vi "Format Table.vi"(8 "button":bool, 9 "clear":bool, 10 "BotPose":cluster{"X":dbl, "Y":dbl}, 11 "Insta360 Pose":cluster{"X":dbl, "Y":dbl}) -> (0 "Points Info for Plot":cluster{dbl[], dbl[], dbl[], dbl[]}, 1 "BoolText.Text":string, 2 "Numeric out":sgl, 3 "Array":string[][](array[string]))   [LabVIEW 2025]
uses:
  d5bf1515-77e7-4290-83ff-5f447d93a6cc.vi
  <vilib>/vision/NI_Vision_Development_Module.lvlib
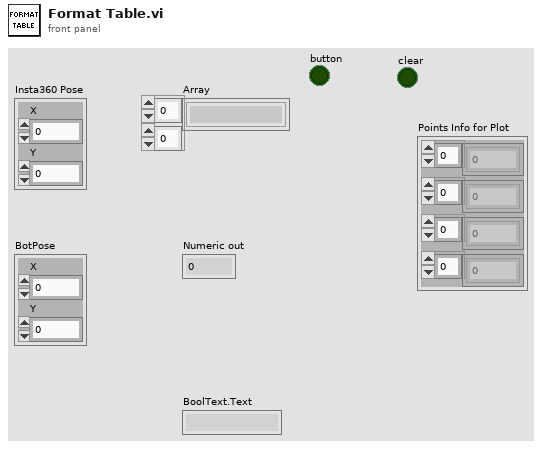
[diagram p1: front panel]
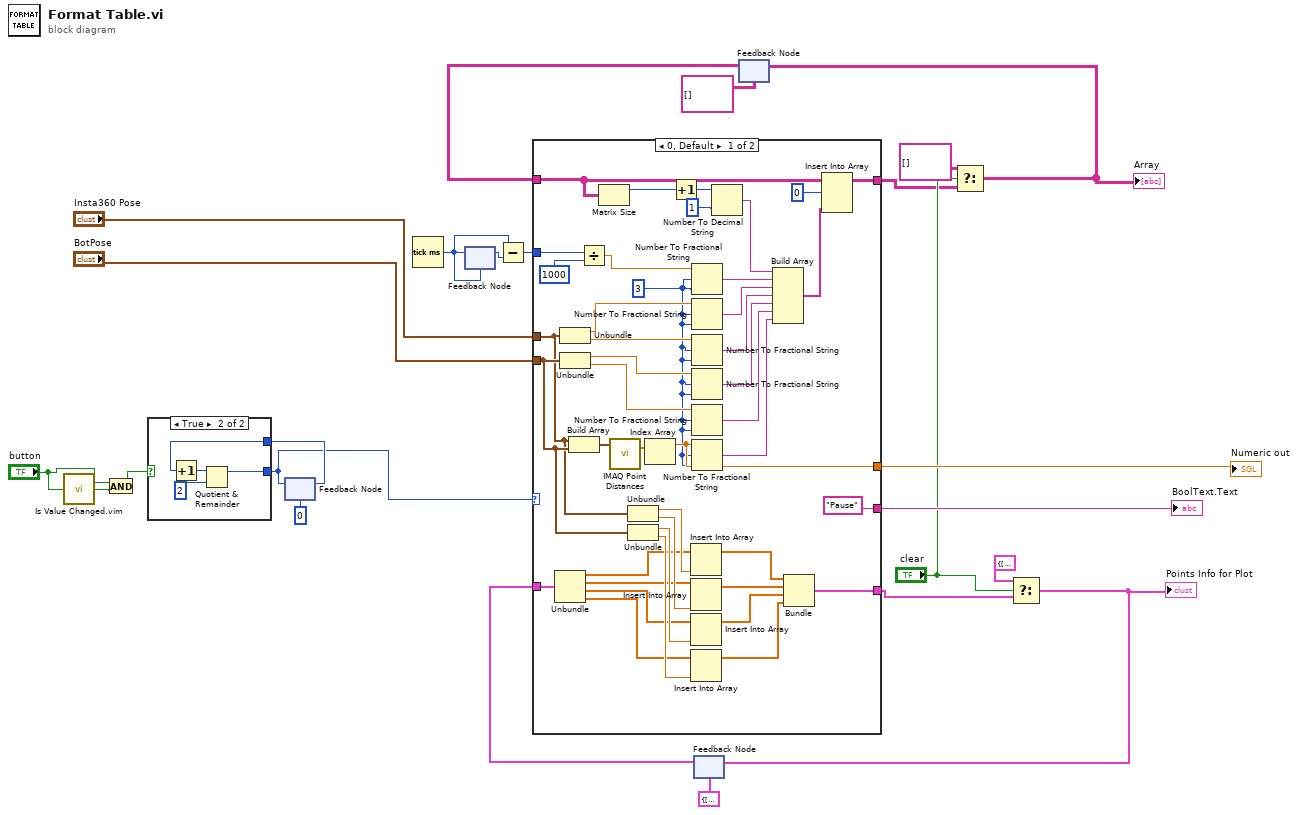
[diagram p0: block diagram]
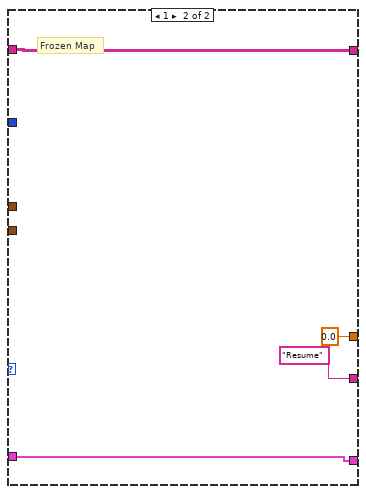
[diagram p3: hidden frame]
diagram:
  n1 = call "Is Value Changed.vim"("value"="button") -> ("changed or first call?"=w15:bool)
  n2 = And(x="button", y=w15) -> (x .and. y?=w16:bool)
  n3 = feedback #1(u16 0) -> (w17:u16)
  n4 = case shown="True" w16 {
    tunnel: w17 -> [w25 w29]
    tunnel: [w25 w26] -> w14
    frame False {
    }
    frame True {
      n5 = Increment(x=w29) -> (x+1=w28:u16)
      n6 = Quotient & Remainder(x=w28, y=u16 2) -> (x-y*floor(x/y)=w26:u16)  [unwired: 1 out]
    }
  }
  n7 = feedback-in #1(w14) -> ()
  n8 = Tick Count (ms)() -> (millisecond timer value=w2:u32)
  n9 = feedback-in #2(w2) -> ()
  n10 = feedback #2(w2) -> (w1:u32)
  n11 = Subtract(x=w2, y=w1) -> (x-y=w3:u32)
  n12 = feedback #3(cluster{dbl[], dbl[], dbl[], dbl[]} {[], [], [], []}) -> (w12:cluster{dbl[], dbl[], dbl[], dbl[]})
  n13 = feedback #4(string[][] []) -> (w21:string[][])
  n14 = case shown="0, Default" w14 {
    tunnel: ["Pause" ("BoolText.Text") "Resume" ("BoolText.Text")] -> w19
    tunnel: w3 -> [w32 _]
    tunnel: w21 -> [w70 w74]
    tunnel: [w64 w74] -> w6
    tunnel: "Insta360 Pose" -> [w47 _]
    tunnel: "BotPose" -> [w48 _]
    tunnel: [w52 sgl 0.0] -> w22
    tunnel: [w38 w72] -> w10
    tunnel: w12 -> [w37 w72]
    frame 0, Default {
      w51 = i16 3 ("width (-)")
      n15 = Unbundle(w37) -> (w36:dbl[], w35:dbl[], w34:dbl[], w33:dbl[])
      n16 = Unbundle(w47) -> ("X"=w63:dbl, "Y"=w62:dbl)
      n17 = Unbundle(w48) -> ("X"=w61:dbl, "Y"=w60:dbl)
      n18 = Build Array(w47, w48) -> (w59:cluster{"X":dbl, "Y":dbl}[])
      n19 = Divide(x=w32, y=u32 1000) -> (x/y=w30:dbl)
      n20 = Matrix Size(0:w70) -> (1:w69:i32)  [unwired: 1 out]
      n21 = call "IMAQ Point Distances"("Points"=w59) -> ("Distances"=w53:sgl[])  [unwired: 4 in, 1 out]
      n22 = Unbundle(w47) -> ("X"=w43:dbl, "Y"=w44:dbl)
      n23 = Unbundle(w48) -> ("X"=w45:dbl, "Y"=w46:dbl)
      n24 = Index Array(array=w53) -> (element=w52:sgl)  [unwired: 1 in]
      n25 = Increment(x=w69) -> (x+1=w50:i32)
      n26 = Insert Into Array(array=w36, new element=w43) -> (w42:dbl[])  [unwired: 1 in]
      n27 = Insert Into Array(array=w35, new element=w44) -> (w41:dbl[])  [unwired: 1 in]
      n28 = Insert Into Array(array=w34, new element=w45) -> (w40:dbl[])  [unwired: 1 in]
      n29 = Insert Into Array(array=w33, new element=w46) -> (w39:dbl[])  [unwired: 1 in]
      n30 = Number To Fractional String(number=w30, width (-)=w51, precision (6)=w51) -> (F-format string=w68:string)  [unwired: 1 in]
      n31 = Number To Fractional String(number=w63, width (-)=w51, precision (6)=w51) -> (F-format string=w58:string)  [unwired: 1 in]
      n32 = Number To Fractional String(number=w62, width (-)=w51, precision (6)=w51) -> (F-format string=w57:string)  [unwired: 1 in]
      n33 = Number To Fractional String(number=w61, width (-)=w51, precision (6)=w51) -> (F-format string=w56:string)  [unwired: 1 in]
      n34 = Number To Fractional String(number=w60, width (-)=w51, precision (6)=w51) -> (F-format string=w55:string)  [unwired: 1 in]
      n35 = Number To Fractional String(number=w52, width (-)=w51, precision (6)=w51) -> (F-format string=w54:string)  [unwired: 1 in]
      n36 = Number To Decimal String(number=w50, width (-)=i16 1) -> (decimal integer string=w67:string)
      n37 = Build Array(w67, w68, w58, w57, w56, w55, w54) -> (w66:string[])
      n38 = Bundle(w42, w41, w40, w39) -> (w38:cluster{dbl[], dbl[], dbl[], dbl[]})  [unwired: 1 in]
      n39 = Insert Into Array(array=w70, index (row)=0, new element=w66) -> (w64:string[][])  [unwired: 1 in]
    }
    frame 1 {
      # "Frozen Map"
    }
  }
  "Numeric out" <- w22
  "BoolText.Text" <- w19
  n40 = Select(t=string[][] [], s="clear", f=w6) -> (s? t:f=w4:string[][])
  "Array" <- w4
  n41 = feedback-in #4(w4) -> ()
  n42 = Select(t=cluster{dbl[], dbl[], dbl[], dbl[]} {[], [], [], []}, s="clear", f=w10) -> (s? t:f=w8:cluster{dbl[], dbl[], dbl[], dbl[]})
  "Points Info for Plot" <- w8
  n43 = feedback-in #3(w8) -> ()
